vi "MyHostCode 2.vi"() -> ()   [LabVIEW 2017]
doc: "This VI was generated automatically using the FPGA Wizard. You can modify the VI normally."
uses:
  <vilib>/rvi/interface/nirviMethod/nirviMethod.xnode
  <vilib>/rvi/interface/nirviCloseFPGA/nirviCloseFPGA.xnode
  <vilib>/rvi/interface/nirviOpenFPGA/nirviOpenFPGA.xnode
  <vilib>/rvi/interface/nirviReadWriteControl/nirviReadWriteControl.xnode
  <vilib>/rvi/errors/niLvFpgaAdjustHostInterfaceError.vi
  <vilib>/rvi/interface/Simulation/niFpgaSimulationCallBeginRW.vi
  <vilib>/FPGAPlugInAG/Dynamic/niLvFpga_ReadFifo_Dynamic.vi
  <vilib>/rvi/errors/niLvFpgaMergeErrorWithErrorCode.vi
  HostCode.lvlib
  <vilib>/Utility/file.llb/Write To Spreadsheet File (I64).vi
  SerialComm/SerialComm.lvclass
  C:/Program Files (x86)/National Instruments/LabVIEW 2017/examples/Instrument IO/Serial/support/Serial - Settings.ctl
  <vilib>/FPGAPlugInAG/Dynamic/niLvFpga_Reset_Dynamic.vi
  <vilib>/FPGAPlugInAG/Dynamic/niLvFpga_Run_Dynamic.vi
  FPGACode/ECG AF SPI Input.vi
  <vilib>/FPGAPlugInAG/Dynamic/niLvFpga_Close_Dynamic.vi
  FPGACode/Lead Enum.ctl
  Trigger Params.ctl
  FPGACode/Channel Enum.ctl
panel:
  in  "IBP Filter":bool=TRUE
  in  "IBP Offset":fxp<+/-,16,16>
  in  "IBP Scale":fxp<+/-,16,5>=1.0
  in  "Offset":cluster{"X":i16, "Y":i16, "Z":i16}
  in  "Beta IBP":fxp<+/-,32,-16> format="%#_3g"
  out "Pressure Data":T1(array[cluster])
  in  "ECG Gain":u16(ring)=1 items=["1"=1, "2"=2, "3"=3, "4"=4, "6"=0, "8"=5, "12"=6]
  in  "Channel":i32
  in  "Sensis\nECG Scaling":i16=1 min=1 max=100 step=1
  out "Trigger":i16[][](graph)
  in  "Trigger":T2={"Channel"=enum."II", "Threshold"=1000, "d/dt"=FALSE, "Invert"=FALSE}
  in  "High Pass":bool
  out "Loop Time":u32
  in  "Reset":bool
  out "Taps":dbl[](graph)
  out "Weights":dbl[](graph)
  out "WeightSum":fxp<+/-,33,19> format="%.20g"
  out "BetaProduct":fxp<+/-,32,-1> format="%.33g"
  in  "Filter Size":i16=100
  out "Invasive Blood Pressure":i16[][](graph)
  in  "Plot Info":T5={"Element"={"Lead"=enum."I", "Filter"=TRUE}, "Element 2"={"Lead"=enum."II", "Filter"=TRUE}, "Element 3"={"Lead"=enum."III", "Filter"=TRUE}, "Element 4"={"Lead"=enum."aVF", "Filter"=TRUE}, "Element 5"={"Lead"=enum."RA", "Filter"=TRUE}, "Element 6"={"Lead"=enum."LA", "Filter"=TRUE}, "Element 7"={"Lead"=enum."LL", "Filter"=TRUE}, "Element 8"={"Lead"=enum."V1", "Filter"=TRUE}}
  in  "file path (dialog if empty)":path
  in  "Record":bool
  out "Gradients":i16[][](graph)
  in  "ECG Filter":bool=TRUE
  out "ECG":i16[][](graph)
  out "Actual Loop Rate (Ticks)":u32
  in  "Beta":fxp<+/-,32,-16>=1.000088900582341e-11 format="%#_4e"
  out "Late? Latched":bool
  in  "Start":bool
  in  "Loop Rate (Hz)":dbl=10000.0
  out "Calculated Rate (Hz)":dbl
  out "error out":errorcluster
  in  "Global Stop":bool
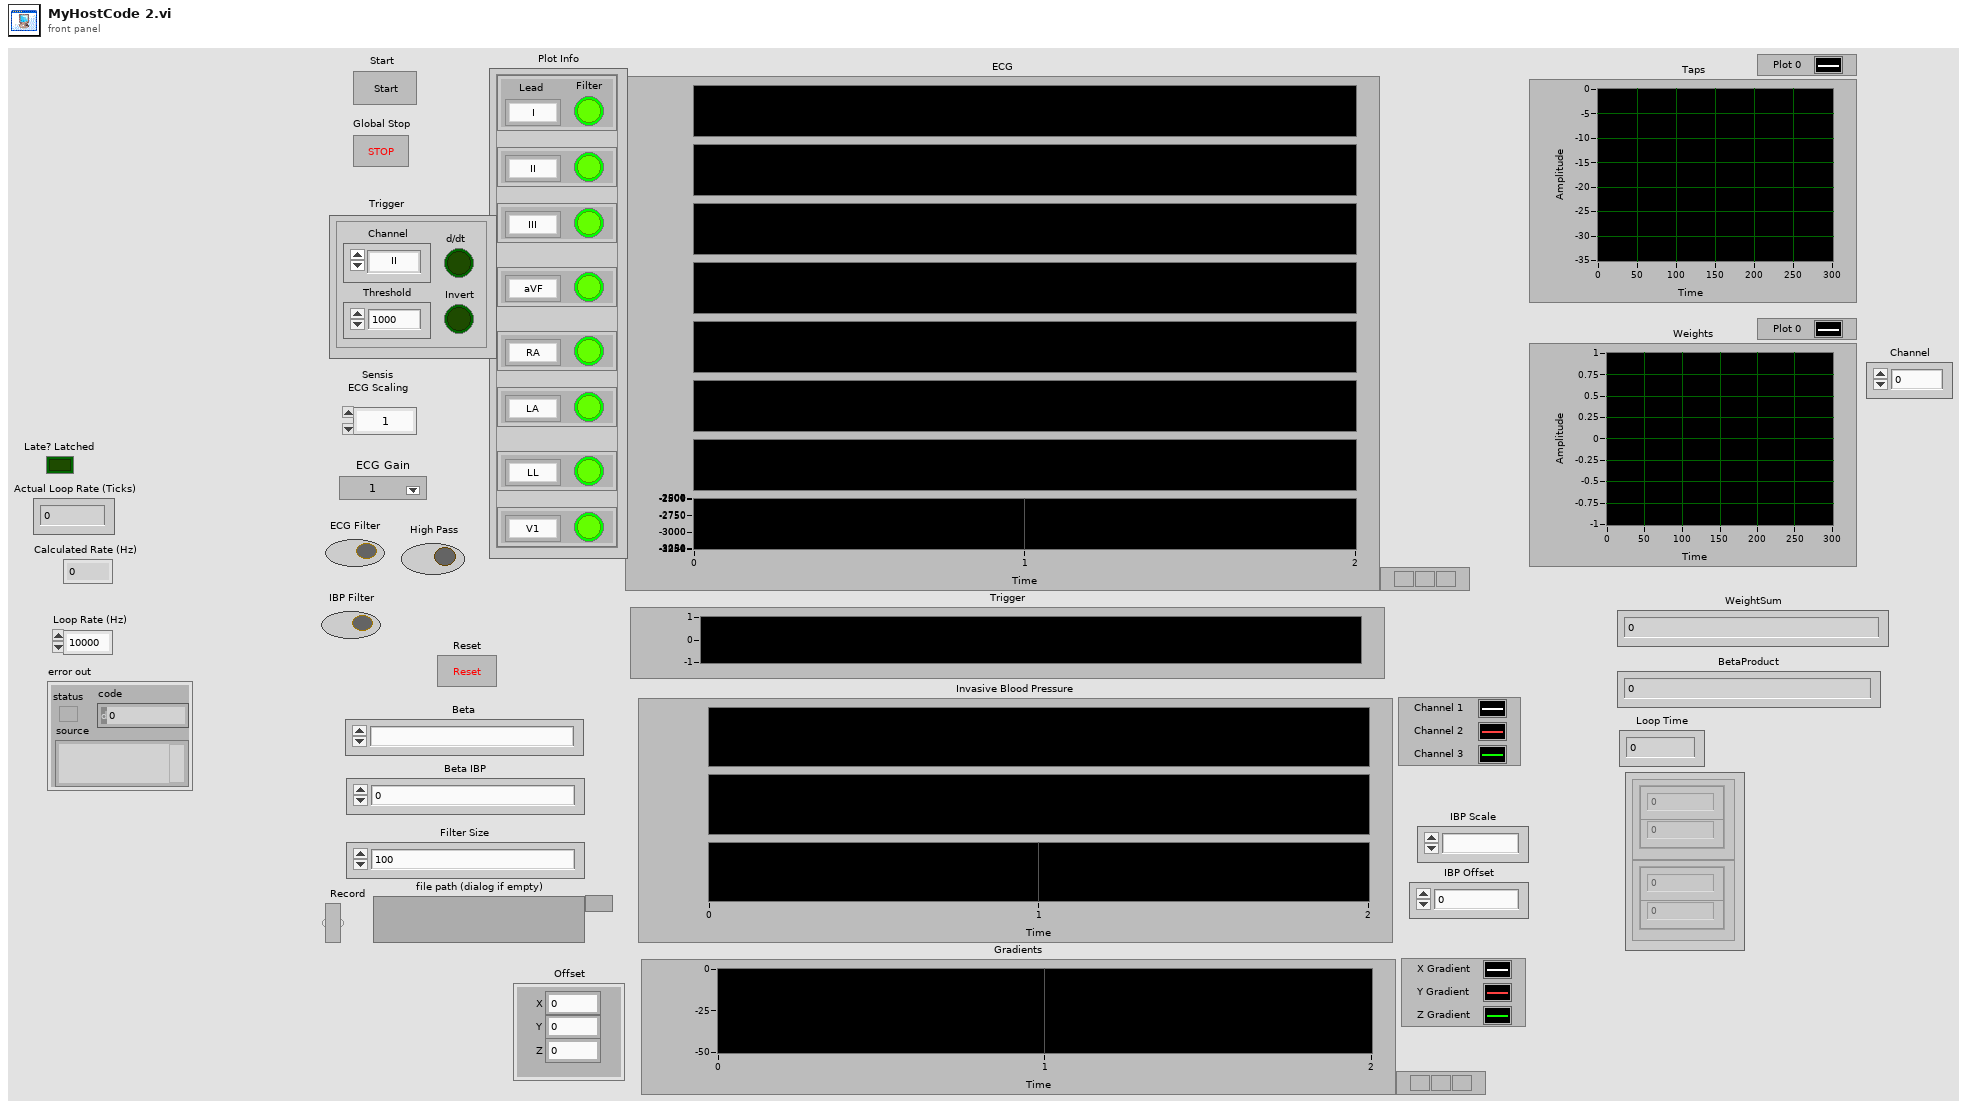
[diagram p1: front panel]
types:
  T1 = cluster{"Numeric Control":dbl, "Numeric Control":dbl}[]
  T2 = typedef "HostCode.lvlib/Trigger Params.ctl" = cluster{"Channel":T3, "Threshold":i16, "d/dt":bool, "Invert":bool}
  T3 = typedef "Channel Enum.ctl" = enum16{"RA", "LA", "LL", "V1", "V2", "V3", "V4", "V5", "V6", "I", "II", "III", "aVR", "aVL", "aVF", "Vw", "IBP1", "IBP2"}
  T4 = typedef "Lead Enum.ctl" = enum16{"RA", "LA", "LL", "V1", "V2", "V3", "V4", "V5", "V6", "I", "II", "III", "aVR", "aVL", "aVF", "Vw"}
  T5 = cluster{"Element":cluster{"Lead":T4, "Filter":bool}, "Element 2":cluster{"Lead":T4, "Filter":bool}, "Element 3":cluster{"Lead":T4, "Filter":bool}, "Element 4":cluster{"Lead":T4, "Filter":bool}, "Element 5":cluster{"Lead":T4, "Filter":bool}, "Element 6":cluster{"Lead":T4, "Filter":bool}, "Element 7":cluster{"Lead":T4, "Filter":bool}, "Element 8":cluster{"Lead":T4, "Filter":bool}}
  T6 = typedef "Serial - Settings.ctl" = cluster{"baud rate":u32, "data bits":u16, "parity":enum16{"None", "Odd", "Even", "Mark", "Space"}, "stop bits":u16, "flow control":u16}
  T7 = typedef "LVOffsetAndMultiplierTypeDef.ctl" = cluster{"Offset":dbl, "Multiplier":dbl}
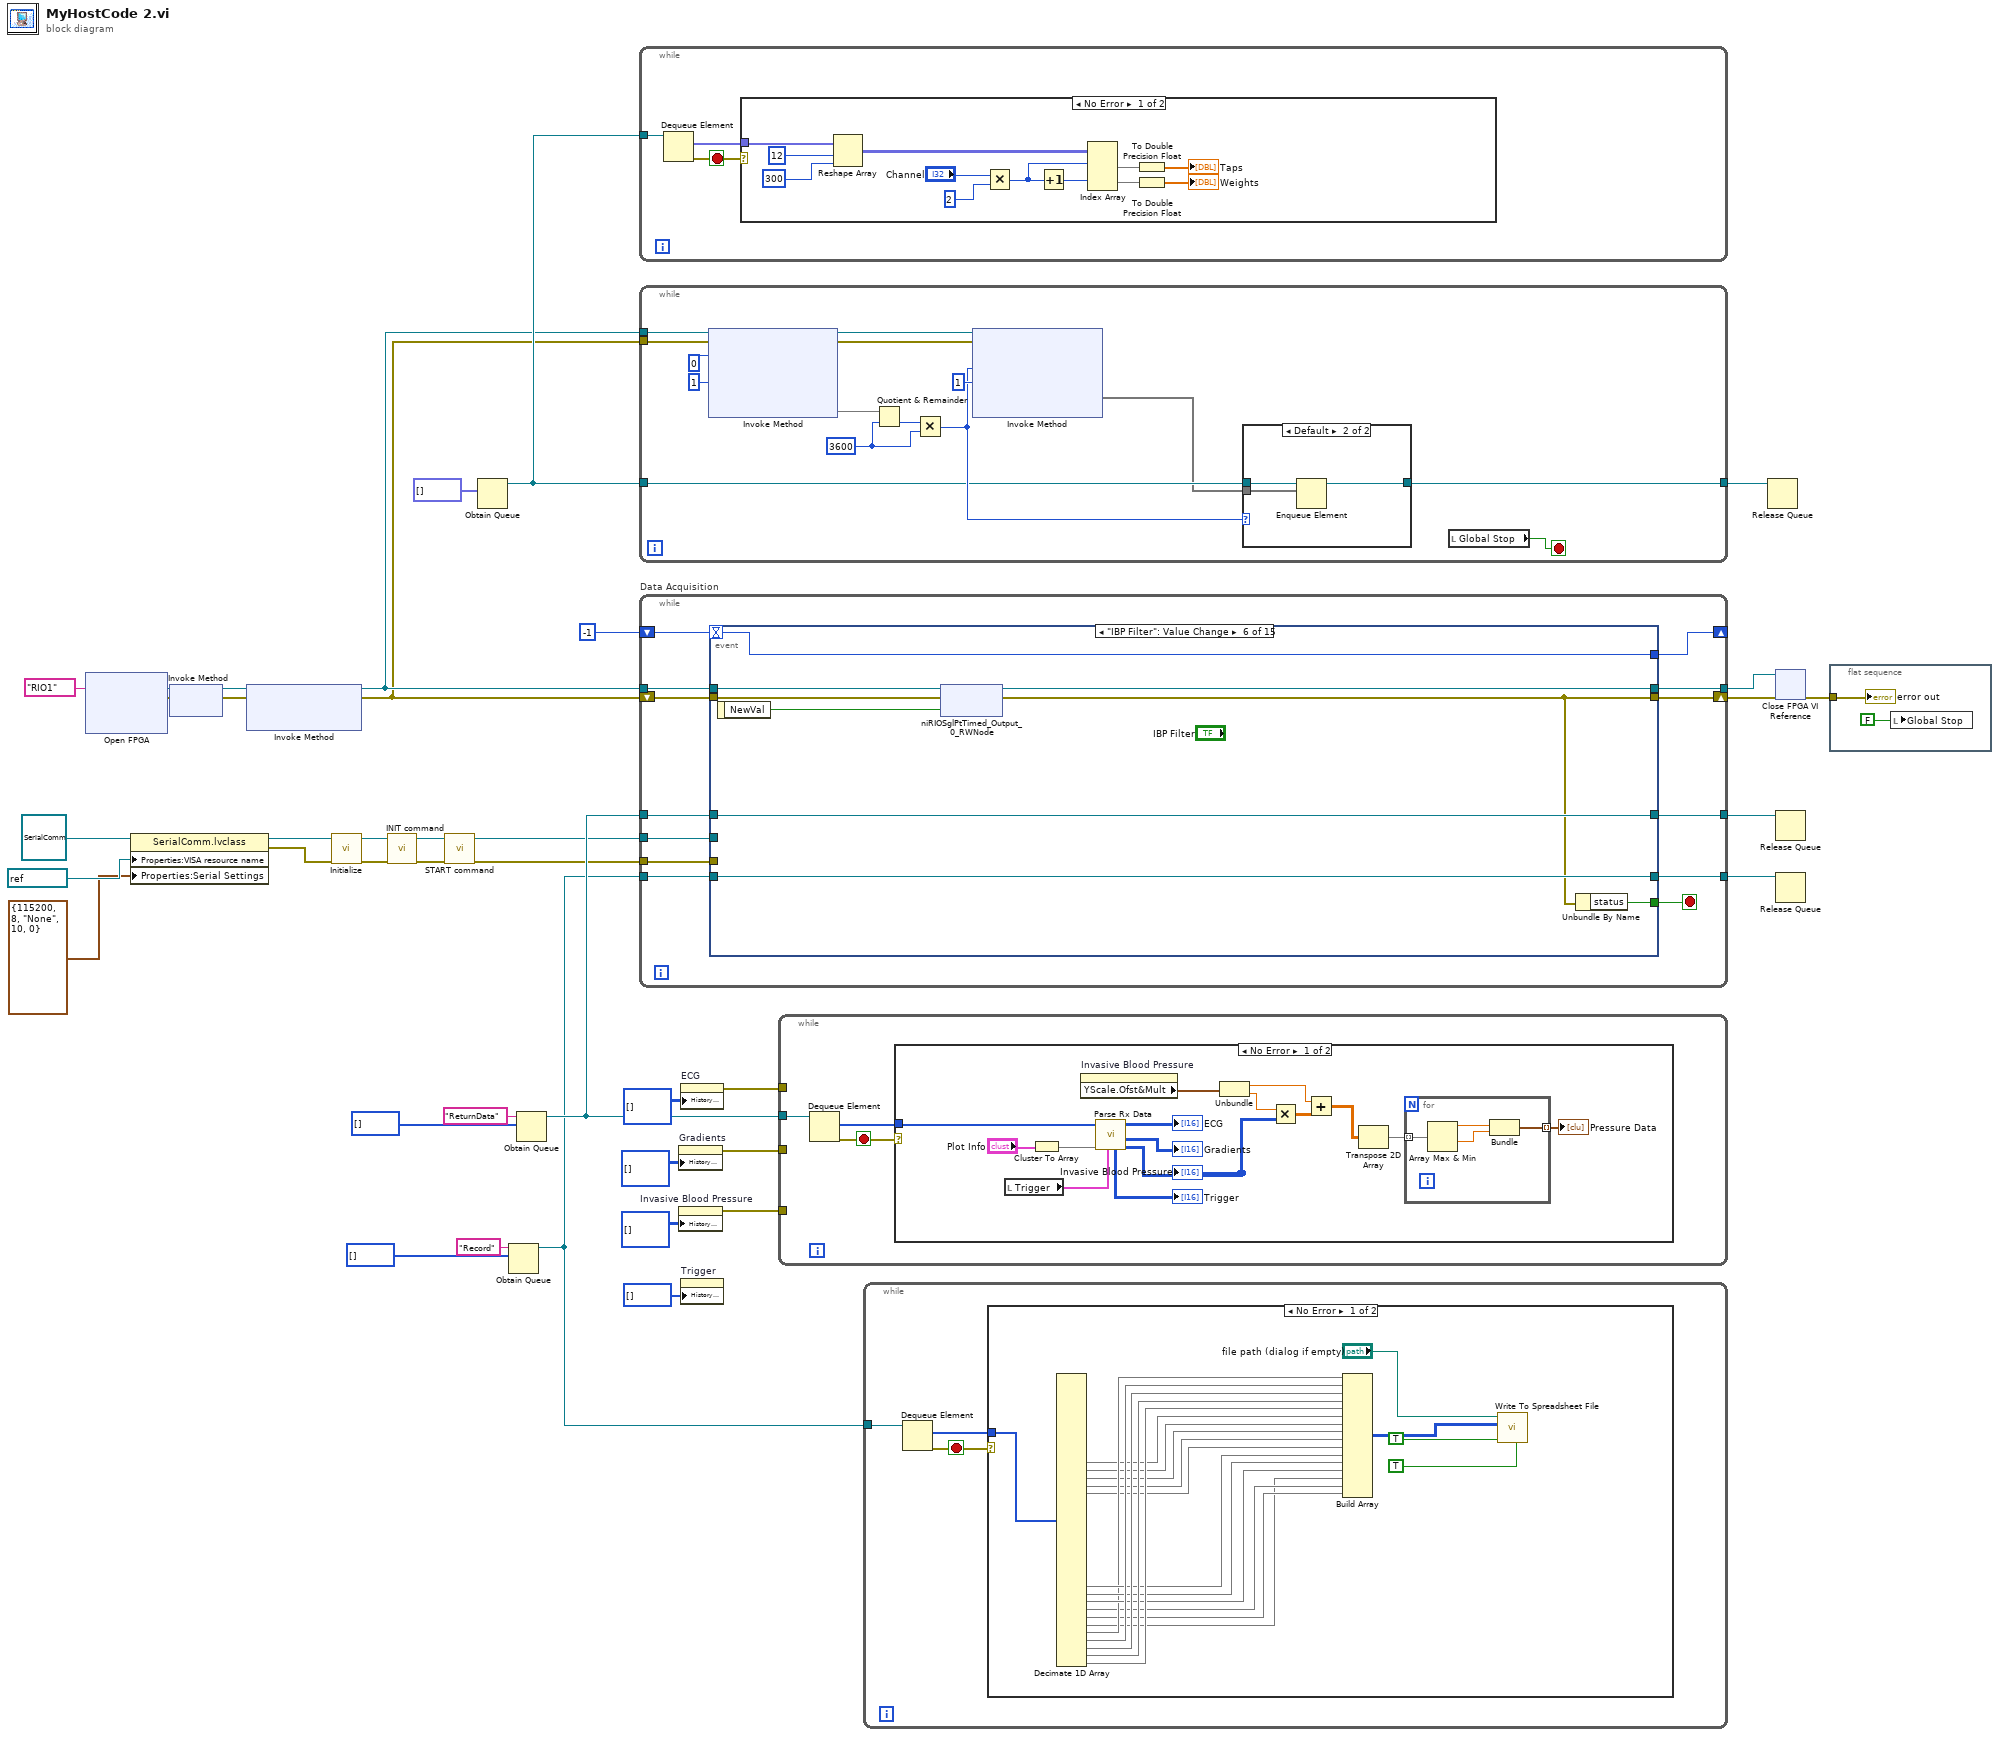
[diagram p0: block diagram]
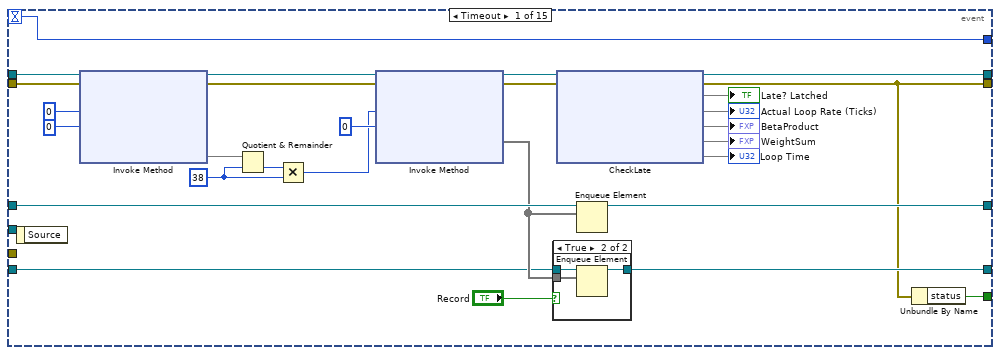
[diagram p2: hidden frame]
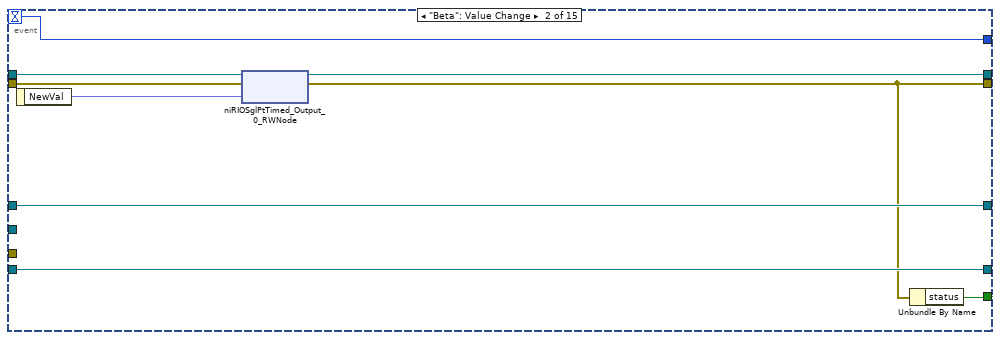
[diagram p4: hidden frame]
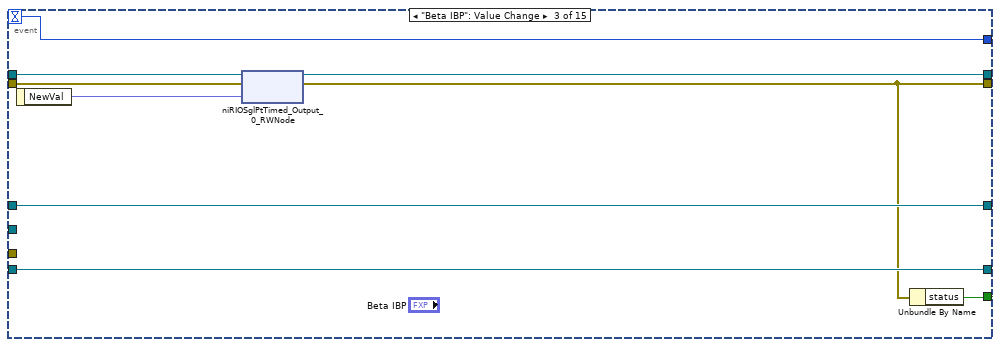
[diagram p5: hidden frame]
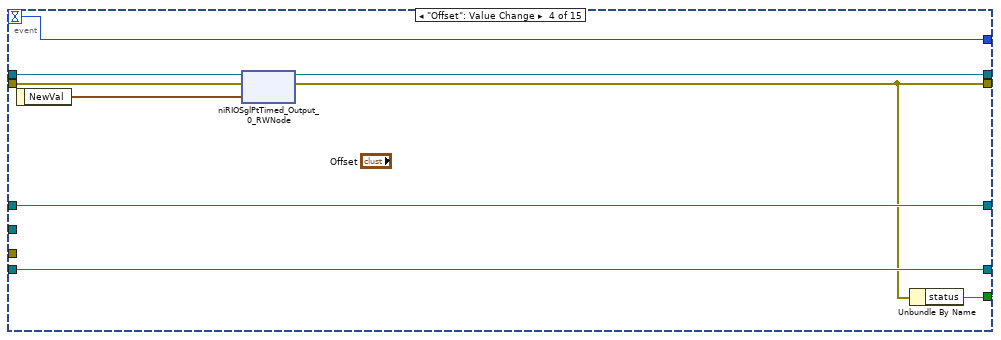
[diagram p6: hidden frame]
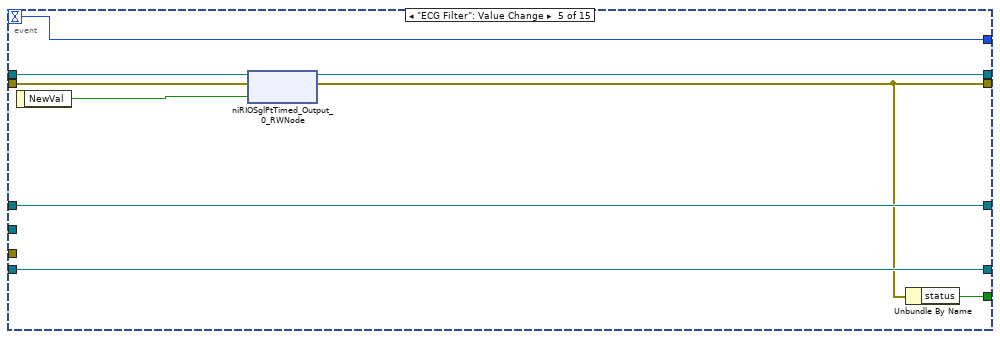
[diagram p7: hidden frame]
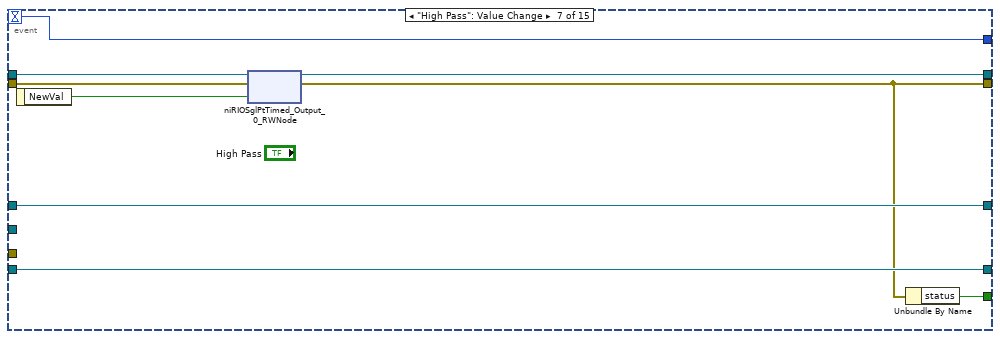
[diagram p8: hidden frame]
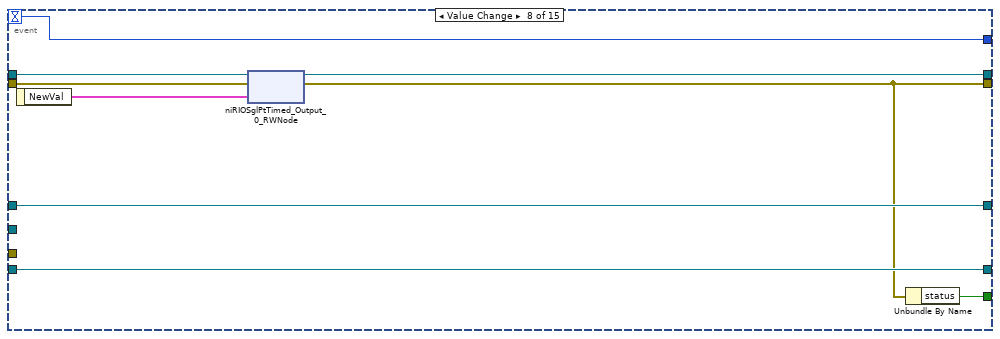
[diagram p9: hidden frame]
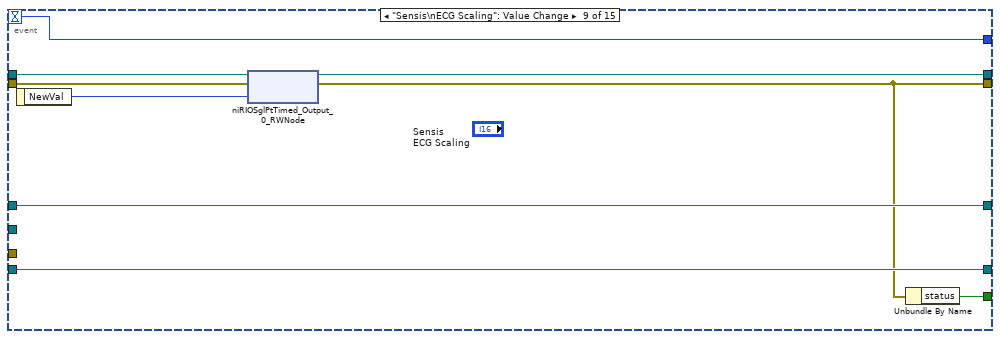
[diagram p10: hidden frame]
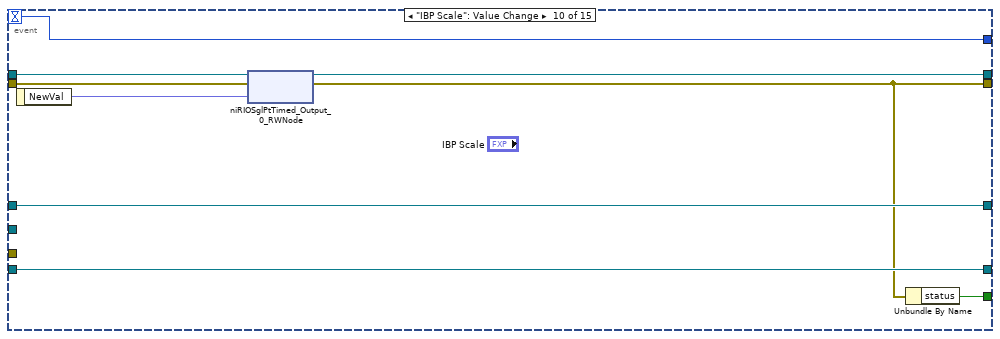
[diagram p11: hidden frame]
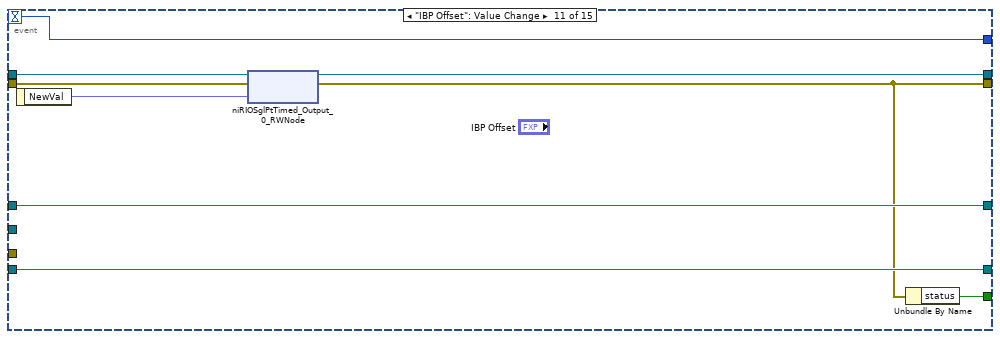
[diagram p12: hidden frame]
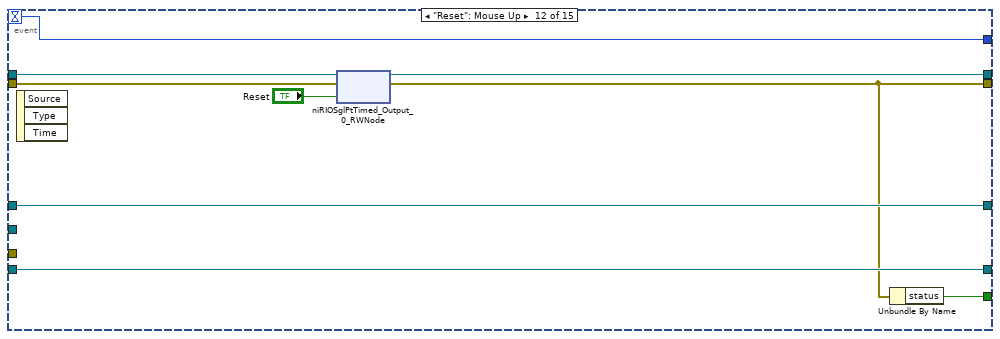
[diagram p13: hidden frame]
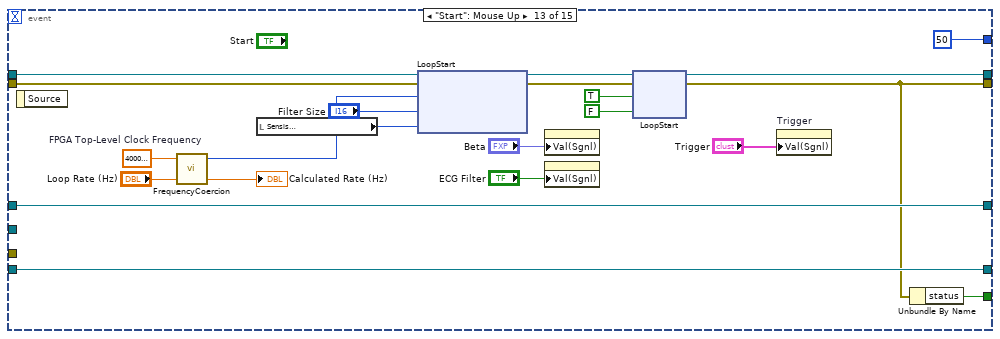
[diagram p14: hidden frame]
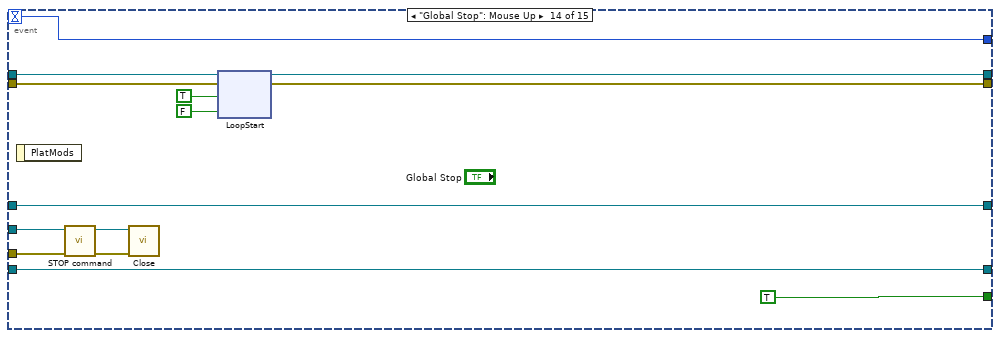
[diagram p15: hidden frame]
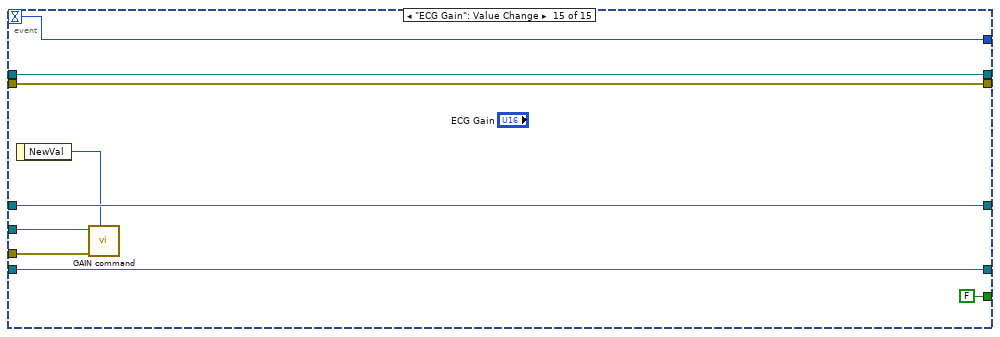
[diagram p16: hidden frame]
diagram:
  n1 = xnode ("Open FPGA")("resource name"=tag "RIO1") -> ("FPGA VI Reference Out"=w39:refnum<k20>, "error out"=w38:errorcluster)  [unwired: 1 in]
  n2 = property class="SerialComm.lvclass"(reference=refnum<class "SerialComm.lvclass"> refnum ("SerialComm.lvclass"), "Properties:VISA resource name"=refnum<visa-resource-name> "COM4" ("VISA resource name"), "Properties:Serial Settings"=T6 {"baud rate"=115200, "data bits"=8, "parity"=enum."None", "stop bits"=10, "flow control"=0} ("Serial Settings")) -> (reference out=w8:refnum<class "SerialComm.lvclass">, error out=w4:errorcluster)  [unwired: 1 in]
  n3 = xnode ("Invoke Method")("FPGA VI Reference In"=w39, "error in"=w38) -> ("FPGA VI Reference Out"=w16:refnum<k20>, "error out"=w40:errorcluster)
  n4 = xnode ("Invoke Method")("FPGA VI Reference In"=w16, "error in"=w40) -> ("FPGA VI Reference Out"=w14:refnum<k20>, "error out"=w13:errorcluster)  [unwired: 1 in]
  n5 = call "Initialize.vi"("Error In"=w4, "SerialComm in"=w8) -> ("Error Out"=w3:errorcluster, "SerialComm out"=w7:refnum<class "SerialComm.lvclass">)  [unwired: 8 in]
  n6 = call "INIT command.vi"("Error In"=w3, "SerialComm in"=w7) -> ("Error Out"=w2:errorcluster, "SerialComm out"=w6:refnum<class "SerialComm.lvclass">)  [unwired: 8 in]
  n7 = call "START command.vi"("Error In"=w2, "SerialComm in"=w6) -> ("Error Out"=w1:errorcluster, "SerialComm out"=w5:refnum<class "SerialComm.lvclass">)  [unwired: 8 in]
  n8 = Obtain Queue(element data type=fxp<+/-,32,16>[] [] ("Data")) -> (queue out=w19:refnum<queue>)  [unwired: 4 in, 2 out]
  n9 = Obtain Queue(name (unnamed)="Record", element data type=i16[] []) -> (queue out=w24:refnum<queue>)  [unwired: 3 in, 2 out]
  n10 = Obtain Queue(name (unnamed)="ReturnData", element data type=i16[] []) -> (queue out=w32:refnum<queue>)  [unwired: 3 in, 2 out]
  n11 = while {
    tunnel: w19 -> [w43]
    stop <- w41 stop-if-true
    n12 = Dequeue Element(queue=w43) -> (element=w42:fxp<+/-,32,16>[], error out=w41:errorcluster)  [unwired: 2 in, 2 out]
    n13 = case shown="No Error" w41 {
      tunnel: w42 -> [w55 _]
      frame No Error {
        n14 = Reshape Array(w55, 12 ("dimension size"), 300 ("dimension size")) -> (w51:fxp<+/-,32,16>[][])
        n15 = Multiply(x="Channel", y=2) -> (x*y=w44:i32)
        n16 = Increment(x=w44) -> (x+1=w45:i32)
        n17 = Index Array(array=w51, index (row) #1=w44, index (row) #2=w45) -> (element #1=w50:fxp<+/-,32,16>[], element #2=w49:fxp<+/-,32,16>[])  [unwired: 2 in]
        n18 = To Double Precision Float(number=w50) -> (double precision float=→"Taps":dbl[])
        n19 = To Double Precision Float(number=w49) -> (double precision float=→"Weights":dbl[])
      }
      frame Error {
      }
    }
  }
  n20 = while {
    tunnel: w14 -> [w70]
    tunnel: w13 -> [w69]
    tunnel: w19 -> [w58]
    tunnel: [w56] -> w18
    stop <- w61 stop-if-true
    w63 = u32 3600 ("y")
    n21 = xnode "Invoke Method"("FPGA VI Reference In"=w70, "error in"=w69, "Number of Elements"=u32 0, "Timeout (ms)"=1) -> ("FPGA VI Reference Out"=w66:refnum<k20>, "error out"=w65:errorcluster, "Elements Remaining"=w62)  [unwired: 1 out]
    n22 = Quotient & Remainder(x=w62, y=w63) -> (floor(x/y)=w64:u32)  [unwired: 1 out]
    n23 = Multiply(x=w64, y=w63) -> (x*y=w59:u32)
    n24 = xnode "Invoke Method"("FPGA VI Reference In"=w66, "error in"=w65, "Number of Elements"=w59, "Timeout (ms)"=1) -> ("Data"=w57:void[])  [unwired: 3 out]
    n25 = case shown="Default" w59 {
      tunnel: w58 -> [w71 w74]
      tunnel: w57 -> [_ w73]
      tunnel: [w71 w72] -> w56
      frame 0 {
      }
      frame Default {
        n26 = Enqueue Element(queue=w74, element=w73) -> (queue out=w72:refnum<queue>)  [unwired: 2 in, 2 out]
      }
    }
    n27 = local read "Global Stop"() -> (w61:bool)
  }
  n28 = while "Data Acquisition" {
    tunnel: w14 -> [w83]
    shift-right: [w87] -> w37
    shift-left: w13 -> [w84]
    tunnel: [w85] -> w35
    tunnel: w32 -> [w82]
    tunnel: [w81] -> w27
    tunnel: w24 -> [w80]
    tunnel: [w79] -> w23
    shift-right: [w77] -> _
    shift-left: -1 -> [w78]
    tunnel: w5 -> [w76]
    tunnel: w1 -> [w75]
    stop <- w86 stop-if-true
    n29 = event shown="[5] \"IBP Filter\": Value Change" {
      selector: _ -> [_ _ _ _ _ _ _ _ _ _ _ _ _ _ _]
      dyn-events: _ -> [_ _ _ _ _ _ _ _ _ _ _ _ _ _ _]
      timeout: w78 -> [w90 w122 w131 w140 w149 w158 w167 w176 w186 w195 w204 w212 _ w246 w260]
      tunnel: [w89 w121 w130 w139 w148 w157 w166 w175 w185 w194 w203 w211 w222 w247 w261] -> w87
      tunnel: [w88 w120 w129 w138 w147 w156 w165 w174 w184 w193 w202 w210 w221 TRUE FALSE ("status")] -> w86
      tunnel: [w115 w126 w135 w144 w153 w162 w171 w180 w189 w198 w207 w216 w227 w248 w262] -> w85
      tunnel: w84 -> [w92 w127 w136 w145 w154 w163 w172 w181 w190 w199 w208 w217 w237 w249 w261]
      tunnel: w83 -> [w93 w128 w137 w146 w155 w164 w173 w182 w191 w200 w209 w218 w238 w250 w262]
      tunnel: w82 -> [w104 w124 w133 w142 w151 w160 w169 w178 w188 w197 w206 w215 w236 w253 w259]
      tunnel: [w100 w124 w133 w142 w151 w160 w169 w178 w188 w197 w206 w215 w236 w253 w259] -> w81
      tunnel: w80 -> [w97 w123 w132 w141 w150 w159 w168 w177 w187 w196 w205 w214 w235 w252 w258]
      tunnel: [w91 w123 w132 w141 w150 w159 w168 w177 w187 w196 w205 w214 w235 w252 w258] -> w79
      tunnel: [w90 w122 w131 w140 w149 w158 w167 w176 w186 w195 w204 w212 50 w246 w260] -> w77
      tunnel: w76 -> [_ _ _ _ _ _ _ _ _ _ _ _ _ w243 w256]
      tunnel: w75 -> [_ _ _ _ _ _ _ _ _ _ _ _ _ w242 w255]
      event Timeout {
        w102 = u32 38 ("y")
        n30 = event-data() -> ()  [unwired: 1 in, 1 out]
        n31 = xnode "Invoke Method"("FPGA VI Reference In"=w93, "error in"=w92, "Number of Elements"=u32 0, "Timeout (ms)"=0) -> ("FPGA VI Reference Out"=w110:refnum<k20>, "error out"=w109:errorcluster, "Elements Remaining"=w108)  [unwired: 1 out]
        n32 = Quotient & Remainder(x=w108, y=w102) -> (floor(x/y)=w103:u32)  [unwired: 1 out]
        n33 = Multiply(x=w103, y=w102) -> (x*y=w101:u32)
        n34 = xnode "Invoke Method"("FPGA VI Reference In"=w110, "error in"=w109, "Number of Elements"=w101, "Timeout (ms)"=0) -> ("FPGA VI Reference Out"=w106:refnum<k20>, "error out"=w105:errorcluster, "Data"=w98:void[])  [unwired: 1 out]
        n35 = case shown="True" "Record" {
          tunnel: w98 -> [_ w119]
          tunnel: w97 -> [w116 w118]
          tunnel: [w116 w117] -> w91
          frame False {
          }
          frame True {
            n36 = Enqueue Element(queue=w118, element=w119) -> (queue out=w117:refnum<queue>)  [unwired: 2 in, 2 out]
          }
        }
        n37 = xnode ("CheckLate")("FPGA VI Reference In"=w106, "error in"=w105) -> ("FPGA VI Reference Out"=w115:refnum<k20>, "error out"=w89:errorcluster, "Late? Latched"=→"Late? Latched", "Actual Loop Rate (Ticks)"=→"Actual Loop Rate (Ticks)", "BetaProduct"=→"BetaProduct", "WeightSum"=→"WeightSum", "Loop Time"=→"Loop Time")
        n38 = Enqueue Element(queue=w104, element=w98) -> (queue out=w100:refnum<queue>)  [unwired: 2 in, 2 out]
        n39 = Unbundle By Name(w89) -> ("status"=w88:bool)
      }
      event "Beta": Value Change {
        n40 = event-data() -> ("NewVal"=w125:fxp<+/-,32,-16>)  [unwired: 1 in]
        n41 = xnode ("niRIOSglPtTimed_Output_0_RWNode")("FPGA VI Reference In"=w128, "error in"=w127, "Beta ECG"=w125) -> ("FPGA VI Reference Out"=w126:refnum<k20>, "error out"=w121:errorcluster)
        n42 = Unbundle By Name(w121) -> ("status"=w120:bool)
      }
      event "Beta IBP": Value Change {
        n43 = event-data() -> ("NewVal"=w134:fxp<+/-,32,-16>)  [unwired: 1 in]
        n44 = xnode ("niRIOSglPtTimed_Output_0_RWNode")("FPGA VI Reference In"=w137, "error in"=w136, "Beta IBP"=w134) -> ("FPGA VI Reference Out"=w135:refnum<k20>, "error out"=w130:errorcluster)
        n45 = Unbundle By Name(w130) -> ("status"=w129:bool)
      }
      event "Offset": Value Change {
        n46 = event-data() -> ("NewVal"=w143:cluster{"X":i16, "Y":i16, "Z":i16})  [unwired: 1 in]
        n47 = xnode ("niRIOSglPtTimed_Output_0_RWNode")("FPGA VI Reference In"=w146, "error in"=w145, "Offset"=w143) -> ("FPGA VI Reference Out"=w144:refnum<k20>, "error out"=w139:errorcluster)
        n48 = Unbundle By Name(w139) -> ("status"=w138:bool)
      }
      event "ECG Filter": Value Change {
        n49 = event-data() -> ("NewVal"=w152:bool)  [unwired: 1 in]
        n50 = xnode ("niRIOSglPtTimed_Output_0_RWNode")("FPGA VI Reference In"=w155, "error in"=w154, "ECG Filter"=w152) -> ("FPGA VI Reference Out"=w153:refnum<k20>, "error out"=w148:errorcluster)
        n51 = Unbundle By Name(w148) -> ("status"=w147:bool)
      }
      event "IBP Filter": Value Change {
        n52 = event-data() -> ("NewVal"=w161:bool)  [unwired: 1 in]
        n53 = xnode ("niRIOSglPtTimed_Output_0_RWNode")("FPGA VI Reference In"=w164, "error in"=w163, "IBP Filter"=w161) -> ("FPGA VI Reference Out"=w162:refnum<k20>, "error out"=w157:errorcluster)
        n54 = Unbundle By Name(w157) -> ("status"=w156:bool)
      }
      event "High Pass": Value Change {
        n55 = event-data() -> ("NewVal"=w170:bool)  [unwired: 1 in]
        n56 = xnode ("niRIOSglPtTimed_Output_0_RWNode")("FPGA VI Reference In"=w173, "error in"=w172, "HPF"=w170) -> ("FPGA VI Reference Out"=w171:refnum<k20>, "error out"=w166:errorcluster)
        n57 = Unbundle By Name(w166) -> ("status"=w165:bool)
      }
      event Value Change {
        n58 = event-data() -> ("NewVal"=w179:T2)  [unwired: 1 in]
        n59 = xnode ("niRIOSglPtTimed_Output_0_RWNode")("FPGA VI Reference In"=w182, "error in"=w181, "Trigger"=w179) -> ("FPGA VI Reference Out"=w180:refnum<k20>, "error out"=w175:errorcluster)
        n60 = Unbundle By Name(w175) -> ("status"=w174:bool)
      }
      event "Sensis\nECG Scaling": Value Change {
        n61 = event-data() -> ("NewVal"=w183:i16)  [unwired: 1 in]
        n62 = xnode ("niRIOSglPtTimed_Output_0_RWNode")("FPGA VI Reference In"=w191, "error in"=w190, "ECG Scale"=w183) -> ("FPGA VI Reference Out"=w189:refnum<k20>, "error out"=w185:errorcluster)
        n63 = Unbundle By Name(w185) -> ("status"=w184:bool)
      }
      event "IBP Scale": Value Change {
        n64 = event-data() -> ("NewVal"=w192:fxp<+/-,16,5>)  [unwired: 1 in]
        n65 = xnode ("niRIOSglPtTimed_Output_0_RWNode")("FPGA VI Reference In"=w200, "error in"=w199, "IBP Scale"=w192) -> ("FPGA VI Reference Out"=w198:refnum<k20>, "error out"=w194:errorcluster)
        n66 = Unbundle By Name(w194) -> ("status"=w193:bool)
      }
      event "IBP Offset": Value Change {
        n67 = event-data() -> ("NewVal"=w201:fxp<+/-,16,16>)  [unwired: 1 in]
        n68 = xnode ("niRIOSglPtTimed_Output_0_RWNode")("FPGA VI Reference In"=w209, "error in"=w208, "IBP Offset"=w201) -> ("FPGA VI Reference Out"=w207:refnum<k20>, "error out"=w203:errorcluster)
        n69 = Unbundle By Name(w203) -> ("status"=w202:bool)
      }
      event "Reset": Mouse Up {
        n70 = event-data() -> ()  [unwired: 1 in, 3 out]
        n71 = xnode ("niRIOSglPtTimed_Output_0_RWNode")("FPGA VI Reference In"=w218, "error in"=w217, "Reset"="Reset") -> ("FPGA VI Reference Out"=w216:refnum<k20>, "error out"=w211:errorcluster)
        n72 = Unbundle By Name(w211) -> ("status"=w210:bool)
      }
      event "Start": Mouse Up {
        w234 = 40000000.0  # FPGA Top-Level Clock Frequency
        n73 = event-data() -> ()  [unwired: 1 in, 1 out]
        n74 = call "FrequencyCoercion.vi"("Loop Rate (Hz)"="Loop Rate (Hz)", "FPGA Top-Level Clock Frequency"=w234) -> ("Actual Rate (Hz)"=→"Calculated Rate (Hz)":dbl, "FPGA Ticks"=w231:u32)  [unwired: 2 in]
        n75 = local read "Sensis\nECG Scaling"() -> (w219:i16)
        n76 = xnode ("LoopStart")("FPGA VI Reference In"=w238, "error in"=w237, "Loop Rate (Ticks)"=w231, "Filter Size"="Filter Size", "ECG Scale"=w219) -> ("FPGA VI Reference Out"=w229:refnum<k20>, "error out"=w228:errorcluster)
        n77 = property on="Beta" class="DigNum (strict)"("Val(Sgnl)"="Beta") -> ()  [unwired: 2 in, 2 out]
        n78 = property on="ECG Filter" class="Bool (strict)"("Val(Sgnl)"="ECG Filter") -> ()  [unwired: 2 in, 2 out]
        n79 = xnode ("LoopStart")("FPGA VI Reference In"=w229, "error in"=w228, "Start"=TRUE ("Start 0"), "Start"=FALSE ("Start 0")) -> ("FPGA VI Reference Out"=w227:refnum<k20>, "error out"=w222:errorcluster)
        n80 = property on="Trigger" class="Clust (strict)"("Val(Sgnl)"="Trigger") -> ()  [unwired: 2 in, 2 out]
        n81 = Unbundle By Name(w222) -> ("status"=w221:bool)
      }
      event "Global Stop": Mouse Up {
        n82 = event-data() -> ()  [unwired: 1 in, 1 out]
        n83 = call "STOP command.vi"("Error In"=w242, "SerialComm in"=w243) -> ("Error Out"=w240:errorcluster, "SerialComm out"=w241:refnum<class "SerialComm.lvclass">)  [unwired: 8 in]
        n84 = call "Close.vi"("Error In"=w240, "SerialComm in"=w241) -> ()  [unwired: 8 in, 2 out]
        n85 = xnode ("LoopStart")("FPGA VI Reference In"=w250, "error in"=w249, "Stop"=TRUE ("stop"), "Stop"=FALSE ("stop")) -> ("FPGA VI Reference Out"=w248:refnum<k20>, "error out"=w247:errorcluster)
      }
      event "ECG Gain": Value Change {
        n86 = event-data() -> ("NewVal"=w254:u16)  [unwired: 1 in]
        n87 = call "GAIN command.vi"("Ring"=w254, "Error In"=w255, "SerialComm in"=w256) -> ()  [unwired: 7 in, 2 out]
      }
    }
  }
  n88 = property on="Gradients" class="WFChart (strict)"("History Data"=i16[][] []) -> (error out=w29:errorcluster)  [unwired: 2 in, 1 out]
  n89 = property on="Invasive Blood Pressure" class="WFChart (strict)"("History Data"=i16[][] []) -> (error out=w21:errorcluster)  [unwired: 2 in, 1 out]
  n90 = property on="ECG" class="WFChart (strict)"("History Data"=i16[][] []) -> (error out=w30:errorcluster)  [unwired: 2 in, 1 out]
  n91 = property on="Trigger" class="WFChart (strict)"("History Data"=i16[] []) -> ()  [unwired: 2 in, 2 out]
  n92 = while {
    tunnel: w32 -> [w265]
    tunnel: w30 -> [_]
    tunnel: w29 -> [_]
    tunnel: w21 -> [_]
    stop <- w264 stop-if-true
    n93 = Dequeue Element(queue=w265) -> (element=w263:i16[], error out=w264:errorcluster)  [unwired: 2 in, 2 out]
    n94 = case shown="No Error" w264 {
      tunnel: w263 -> [w280 _]
      frame No Error {
        n95 = local read "Trigger"() -> (w277:T2)
        n96 = Cluster To Array(cluster="Plot Info") -> (array=w266:cluster{"Lead":T4, "Filter":bool}[])
        n97 = property on="Invasive Blood Pressure" class="WFChart (strict)"() -> ("YScale.Ofst&Mult"=w272:T7)  [unwired: 2 in, 2 out]
        n98 = call "Parse Rx Data.vi"("Trigger"=w277, "Plot Info"=w266, "Input Data"=w280) -> ("Pressures"=w271:i16[][], "Gradients"=→"Gradients":i16[][], "ECG Data"=→"ECG":i16[][], "Trigger"=→"Trigger":i16[][])  [unwired: 5 in]
        "Invasive Blood Pressure" <- w271
        n99 = Unbundle(w272) -> ("Offset"=w268:dbl, "Multiplier"=w270:dbl)
        n100 = Multiply(x=w270, y=w271) -> (x*y=w269:dbl[][])
        n101 = Add(x=w268, y=w269) -> (x+y=w267:dbl[][])
        n102 = Transpose 2D Array(2D array=w267) -> (transposed array=w273:dbl[][])
        n103 = for {
          tunnel: w273 -> [w284] mode=indexing
          tunnel: [w281] -> w274 mode=indexing
          n104 = Array Max & Min(array=w284) -> (max value=w283:dbl, min value=w282:dbl)  [unwired: 2 out]
          n105 = Bundle(w283, w282) -> (w281:cluster{dbl, dbl})  [unwired: 1 in]
        }
        "Pressure Data" <- w274
      }
      frame Error {
      }
    }
  }
  n106 = while {
    tunnel: w24 -> [w285]
    stop <- w287 stop-if-true
    n107 = Dequeue Element(queue=w285) -> (element=w286:i16[], error out=w287:errorcluster)  [unwired: 2 in, 2 out]
    n108 = case shown="No Error" w287 {
      tunnel: w286 -> [w305 _]
      frame No Error {
        n109 = Decimate 1D Array(w305) -> (w295:i16[], w294:i16[], w293:i16[], w292:i16[], w291:i16[], w298:i16[], w299:i16[], w300:i16[], w289:i16[], w290:i16[], w288:i16[], w296:i16[], w304:i16[], w303:i16[], w302:i16[], w301:i16[])  [unwired: 22 out]
        n110 = Build Array(w296, w304, w303, w302, w301, w295, w294, w293, w292, w291, w298, w299, w300, w288, w289, w290) -> (w297:i16[][])
        n111 = call-poly <vilib>:"Write To Spreadsheet File.vi"("transpose? (no:F)"=TRUE, "append to file? (new file:F)"=TRUE, "2D data"=w297, "file path (dialog if empty)"="file path (dialog if empty)") -> ()  [unwired: 4 in, 1 out]
      }
      frame Error {
      }
    }
  }
  n112 = Release Queue(queue=w18) -> ()  [unwired: 2 in, 3 out]
  n113 = xnode ("Close FPGA VI Reference")("FPGA VI Reference In"=w35, "error in"=w37) -> ("error out"=w36:errorcluster)
  n114 = Release Queue(queue=w27) -> ()  [unwired: 2 in, 3 out]
  n115 = Release Queue(queue=w23) -> ()  [unwired: 2 in, 3 out]
  n116 = flat-sequence {
    tunnel: w36 -> [w310]
    frame #0 {
      n117 = local write "Global Stop"(FALSE ("Global Stop")) -> ()
      "error out" <- w310
    }
  }
